vi "Dot.vi"(0 "Dot in":refnum<class "Dot.lvclass">, 5 "id":i32, 7 "x":i32, 9 "y":i32, 11 "error in (no error)":errorcluster) -> (4 "Dot out":refnum<class "Dot.lvclass">, 15 "error out":errorcluster)   [LabVIEW 2017, in "Dot.lvclass"]
uses:
  Dot.lvclass
  Dot.lvclass/Dot.ctl
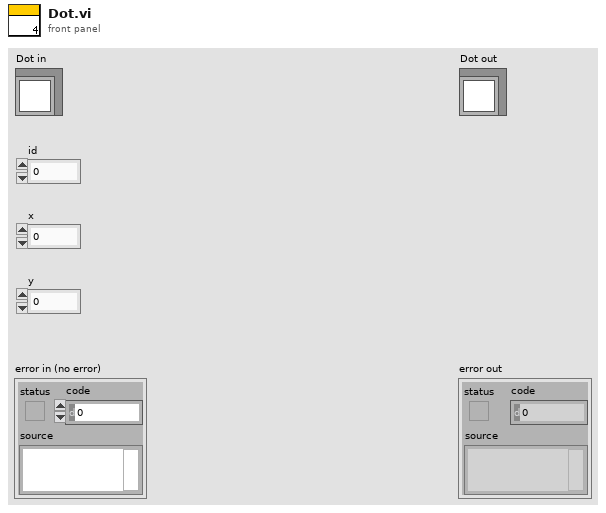
[diagram p1: front panel]
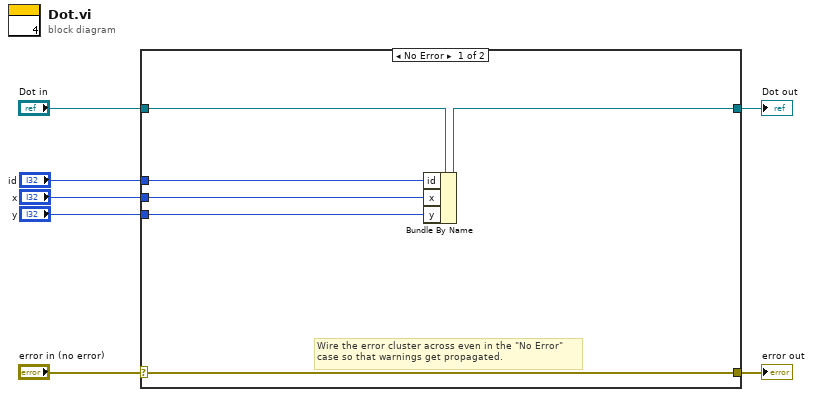
[diagram p0: block diagram]
diagram:
  n1 = case shown="No Error" "error in (no error)" {
    selector: "error in (no error)" -> [w12 w15]
    tunnel: [w12 w15] -> w6
    tunnel: [w11 w14] -> w4
    tunnel: "Dot in" -> [w13 w14]
    tunnel: "id" -> [w10 _]
    tunnel: "x" -> [w9 _]
    tunnel: "y" -> [w8 _]
    frame No Error {
      # "Wire the error cluster across even in the \"No Error\"\ncase so that warnings get propagated."
      n2 = Bundle By Name(cluster=w13, "id"=w10, "x"=w9, "y"=w8) -> (w11:refnum<class "Dot.lvclass">)
    }
    frame Error {
    }
  }
  "error out" <- w6
  "Dot out" <- w4
